vi "Rising Edge Detector with Data Valid.vi"(9 "Data Valid":bool, 10 "signal":bool) -> (2 "edge detected":bool)   [LabVIEW 2014]
panel:
  # "Copyright 2014 Vidrio Technologies\nScanImage 5 software is licensed under the Apache License, Version 2.0 (the \"License\"); you may not use any files contained\nwithin the ScanImage 5 release except in compliance with the License. You may obtain a copy of the License at\n http://www.apache.org/licenses/LICENSE-2.0\nUnless required by applicable law or agreed to in writing, software distributed under the License is distributed on an\n\"AS IS\" BASIS, WITHOUT WARRANTIES OR CONDITIONS OF ANY KIND, either express or implied. See the License for the\n specific language governing permissions and limitations under the License."
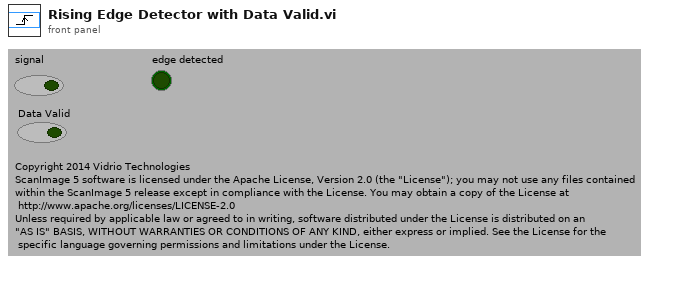
[diagram p1: front panel]
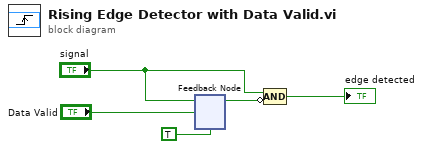
[diagram p0: block diagram]
diagram:
  n1 = feedback-in #1("signal", "Data Valid") -> ()
  n2 = feedback #1(TRUE) -> (w4:bool)
  n3 = Compound Arithmetic op=AND("signal", invert w4) -> (→"edge detected":bool)
